vi "CAN 6 SPARK MAX Motor Set PIDF with Gearing.vi"(9 "PIDF gains Low Gear":T1, 10 "PIDF gains High Gear":T1, 11 "TalonSRX6MotorRef":T2) -> (3 "TalonSRX6MotorRef":T2)   [LabVIEW 2018]
uses:
  SPARKMAX6Motor.ctl
  <vilib>/Rock Robotics/WPI/MotorControl/WPI_MotorControlDeviceRef.ctl
  <vilib>/Rock Robotics/WPI/MotorControl/WPI_MotorControlType.ctl
  <vilib>/Rock Robotics/SystemInterfaces/DIO/FPGA_DIOPWMChannel.ctl
  <vilib>/Rock Robotics/WPI/PWM/WPI_PWMDeadband.ctl
  <vilib>/Rock Robotics/SystemInterfaces/DIO/FPGA_DIOChannel.ctl
panel:
  in  "Max Output":dbl=1.0
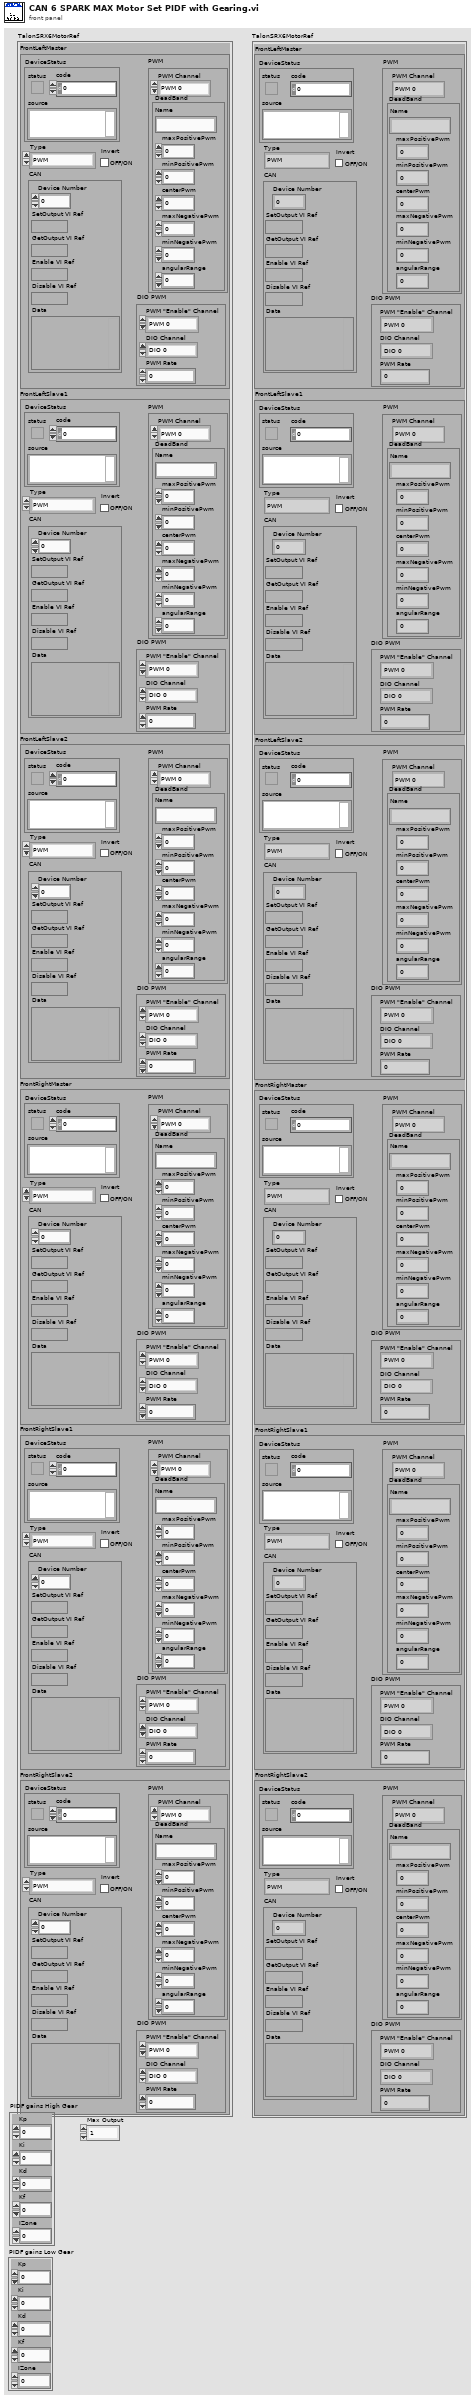
[diagram p1: front panel]
types:
  T1 = cluster{"Kp":dbl, "Ki":dbl, "Kd":dbl, "Kf":dbl, "IZone":dbl}
  T2 = typedef "SPARKMAX6Motor.ctl" = cluster{"FrontLeftMaster":T3, "FrontLeftSlave1":T3, "FrontLeftSlave2":T3, "FrontRightMaster":T3, "FrontRightSlave1":T3, "FrontRightSlave2":T3}
  T3 = typedef "WPI_MotorControlDeviceRef.ctl" = cluster{"DeviceStatus":errorcluster, "Type":T4, "PWM":cluster{"PWM Channel":T5, "DeadBand":T6}, "CAN":cluster{"Device Number":u8, "SetOutput VI Ref":variant, "GetOutput VI Ref":variant, "Enable VI Ref":variant, "Disable VI Ref":variant, "Data":variant}, "Invert":bool, "DIO PWM":cluster{"PWM \"Enable\" Channel":T5, "DIOChannel":T7, "PWM Rate":dbl}}
  T4 = typedef "WPI_MotorControlType.ctl" = enum16{"PWM", "CAN", "DIO PWM"}
  T5 = typedef "FPGA_DIOPWMChannel.ctl" = enum8{"PWM 0", "PWM 1", "PWM 2", "PWM 3", "PWM 4", "PWM 5", "PWM 6", "PWM 7", "PWM 8", "PWM 9", "PWM MXP 0", "PWM MXP 1", "PWM MXP 2", "PWM MXP 3", "PWM MXP 4", "PWM MXP 5", "PWM MXP 6", "PWM MXP 7", "PWM MXP 8", "PWM MXP 9", "Invalid"}
  T6 = typedef "WPI_PWMDeadband.ctl" = cluster{"Name":string, "maxPositivePwm":i32, "minPositivePwm":i32, "centerPwm":i32, "maxNegativePwm":i32, "minNegativePwm":i32, "angularRange":u16}
  T7 = typedef "FPGA_DIOChannel.ctl" = enum8{"DIO 0", "DIO 1", "DIO 2", "DIO 3", "DIO 4", "DIO 5", "DIO 6", "DIO 7", "DIO 8", "DIO 9", "DIO MXP 0", "DIO MXP 1", "DIO MXP 2", "DIO MXP 3", "DIO MXP 4", "DIO MXP 5", "DIO MXP 6", "DIO MXP 7", "DIO MXP 8", "DIO MXP 9", "DIO MXP 10", "DIO MXP 11", "DIO MXP 12", "DIO MXP 13", "DIO MXP 14", "DIO MXP 15", "SPI Port CS1", "SPI Port CS2", "SPI Port CS3", "SPI Port MISO", "SPI Port MOSI", "Invalid"}
  T8 = cluster{"P Gain":dbl, "I Gain":dbl, "D Gain":dbl, "F Gain":dbl, "I Zone":dbl, "Min Output":dbl, "Max Output":dbl}
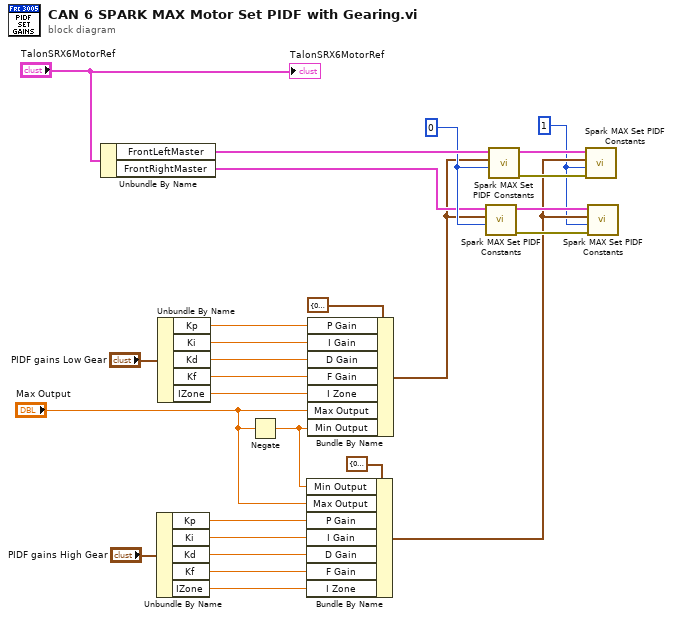
[diagram p0: block diagram]
diagram:
  w3 = 0 ("PIDF Slot")
  w4 = 1 ("PIDF Slot")
  n1 = Unbundle By Name("TalonSRX6MotorRef") -> ("FrontLeftMaster"=w10:T3, "FrontRightMaster"=w2:T3)
  n2 = Unbundle By Name("PIDF gains High Gear") -> ("Kp"=w14:dbl, "Ki"=w15:dbl, "Kd"=w16:dbl, "Kf"=w17:dbl, "IZone"=w18:dbl)
  n3 = Unbundle By Name("PIDF gains Low Gear") -> ("Kp"=w24:dbl, "Ki"=w23:dbl, "Kd"=w22:dbl, "Kf"=w20:dbl, "IZone"=w21:dbl)
  n4 = Negate(x="Max Output") -> (-x=w12:dbl)
  n5 = Bundle By Name(cluster=T8 {"P Gain"=0.0, "I Gain"=0.0, "D Gain"=0.0, "F Gain"=0.0, "I Zone"=0.0, "Min Output"=-1.0, "Max Output"=1.0} ("PID Constants"), "Min Output"=w12, "Max Output"="Max Output", "P Gain"=w14, "I Gain"=w15, "D Gain"=w16, "F Gain"=w17, "I Zone"=w18) -> (w5:T8)
  n6 = Bundle By Name(cluster=T8 {"P Gain"=0.0, "I Gain"=0.0, "D Gain"=0.0, "F Gain"=0.0, "I Zone"=0.0, "Min Output"=-1.0, "Max Output"=1.0} ("PID Constants"), "P Gain"=w24, "I Gain"=w23, "D Gain"=w22, "F Gain"=w20, "I Zone"=w21, "Max Output"="Max Output", "Min Output"=w12) -> (w1:T8)
  n7 = call <vilib>:"Spark MAX Set PIDF Constants.vi"("PIDF Slot"=w3, "PID Constants"=w1, "MotorControlDeviceRef"=w2) -> ("error out"=w6:errorcluster, "MotorControlDeviceRef"=w7:T3)  [unwired: 7 in]
  n8 = call <vilib>:"Spark MAX Set PIDF Constants.vi"("PIDF Slot"=w3, "PID Constants"=w1, "MotorControlDeviceRef"=w10) -> ("error out"=w9:errorcluster, "MotorControlDeviceRef"=w8:T3)  [unwired: 7 in]
  n9 = call <vilib>:"Spark MAX Set PIDF Constants.vi"("error in"=w9, "PIDF Slot"=w4, "PID Constants"=w5, "MotorControlDeviceRef"=w8) -> ()  [unwired: 6 in, 2 out]
  n10 = call <vilib>:"Spark MAX Set PIDF Constants.vi"("error in"=w6, "PIDF Slot"=w4, "PID Constants"=w5, "MotorControlDeviceRef"=w7) -> ()  [unwired: 6 in, 2 out]
  "TalonSRX6MotorRef" <- "TalonSRX6MotorRef"
